vi "Bob.vi"() -> ()   [LabVIEW 2013]
panel:
  in  "Tabs":enum32{"1", "2", "3"}(tab)=enum."2"
  in  "SortearBase":bool
  out "Bases e Estados":string[][](table)=[["", "1", "2", "3", "4", "5", "6", "7", "8", "9", "10", "11", "12", "13", "14", "15", "16", "17", "18", "19", "20"], ["Base", "", "", "", "", "", "", "", "", "", "", "", "", "", "", "", "", "", "", "", ""], ["Estado", "", "", "", "", "", "", "", "", "", "", "", "", "", "", "", "", "", "", "", ""], ["Polarização", "", "", "", "", "", "", "", "", "", "", "", "", "", "", "", "", "", "", "", ""]] caption="Sorteio dos estados para leitura"
  out "Figura":u16(ring)
  in  "MoedaBase":u16(ring)
  in  "Iniciar Calibragem":bool
  in  "Waveform Chart":dbl(graph)
  in  "Coletar medida":bool
  out "Ring":u16(ring) items=["nulo", "nulo", "V", "H", "nulo", "A", "D"]
  in  "ContadorBase":u8=1 min=1
  # "II Semana de Física Experimental"
  # "Criptografia Quântica"
  # "Bob"
  # "Laboratório de Óptica Quântica"
  # "UFRJ"
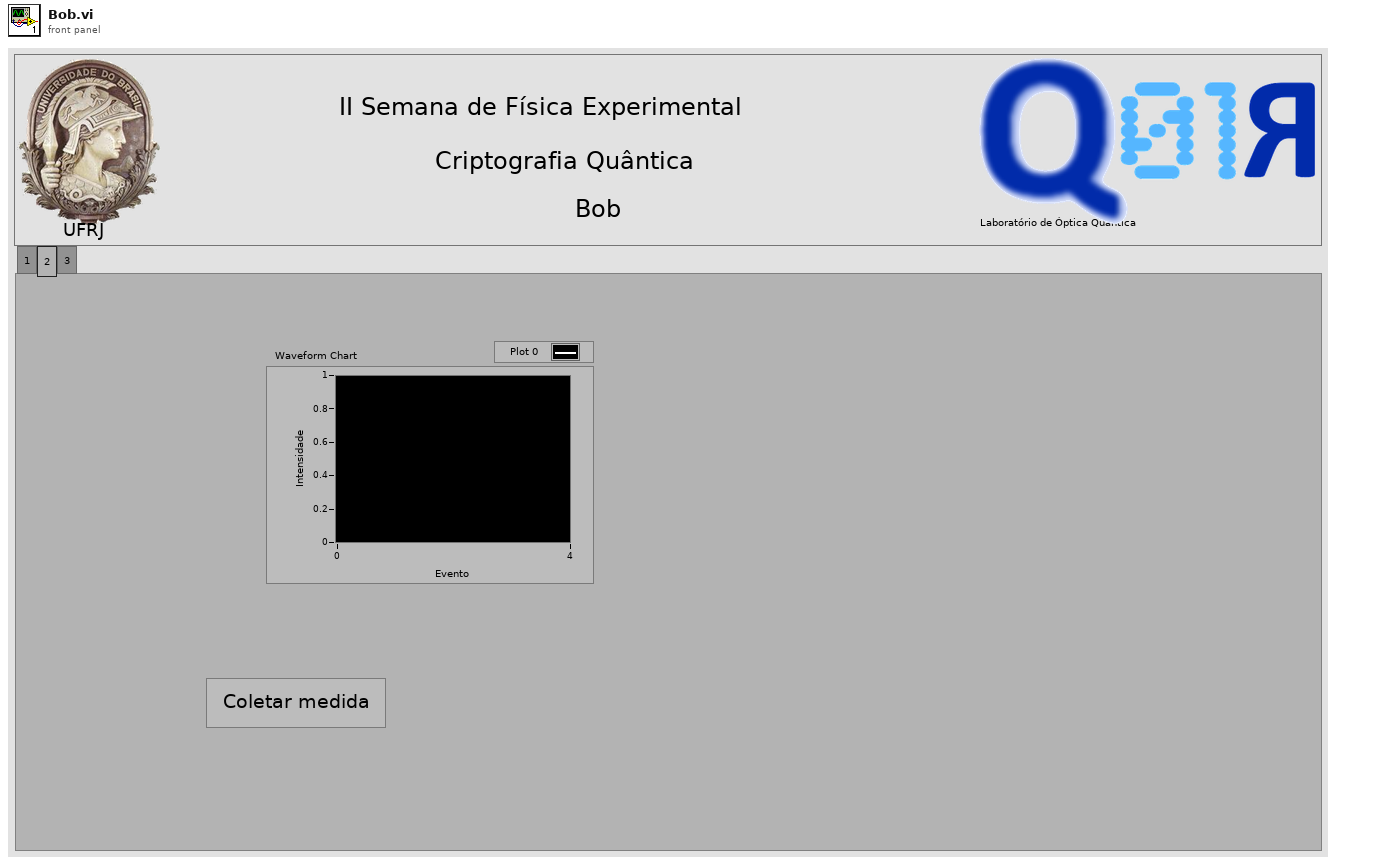
[diagram p1: front panel]
types:
  T1 = enum32{"Page Enabled", "Page Disabled", "Page Disabled & Grayed"}[]
  T2 = enum8{"Enabled", "Disabled", "Disabled and Grayed Out"}
  T3 = enum16{"BCBR", "BC", "BC0", "BC1", "BR", "BR0", "BR1"}
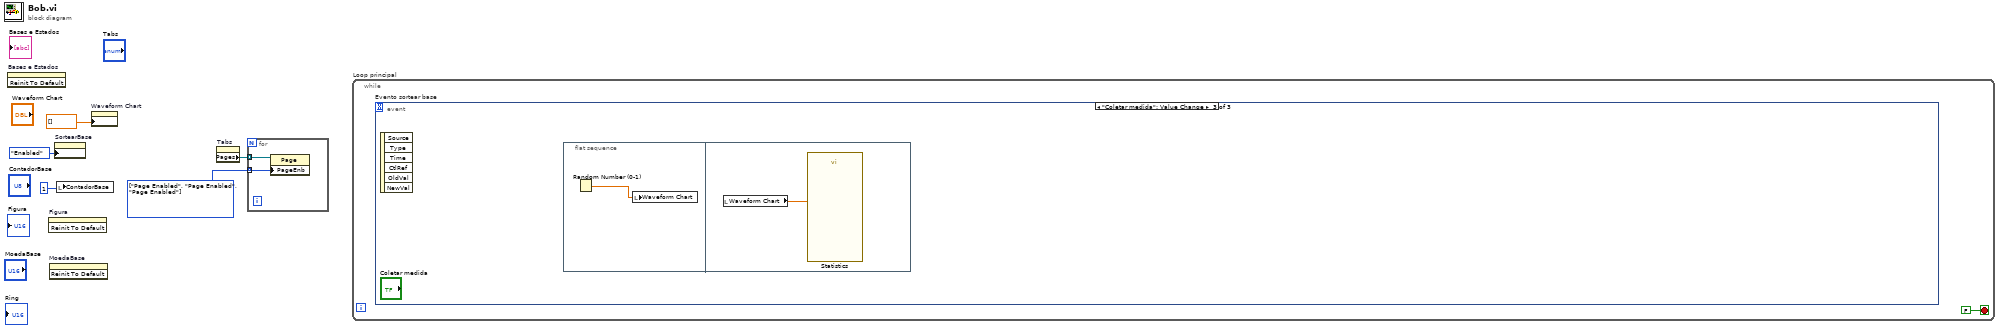
[diagram p0: block diagram]
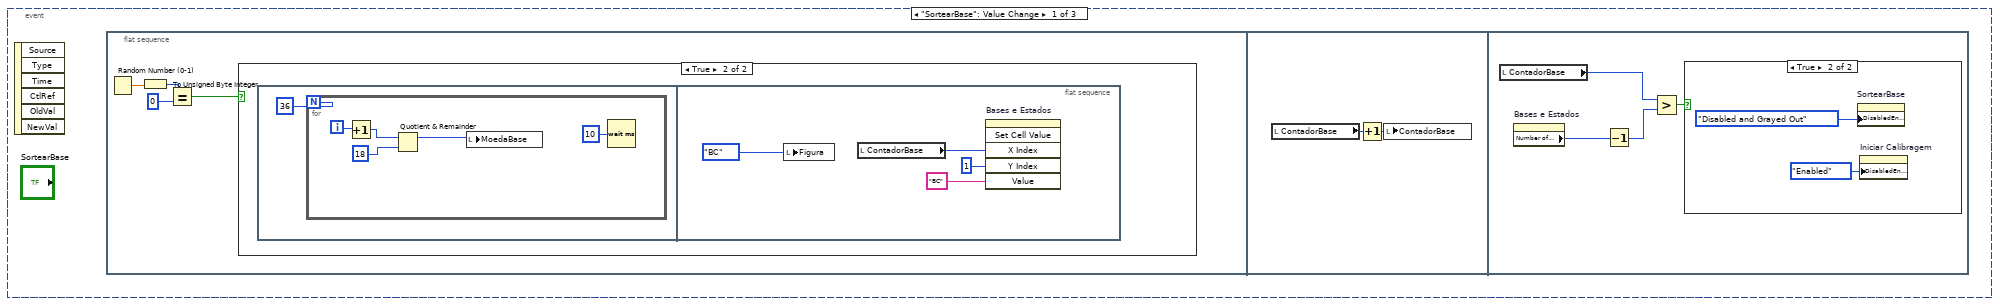
[diagram p2: hidden frame]
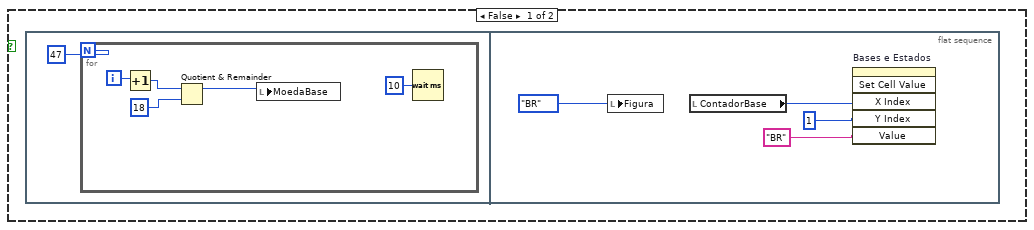
[diagram p3: hidden frame]
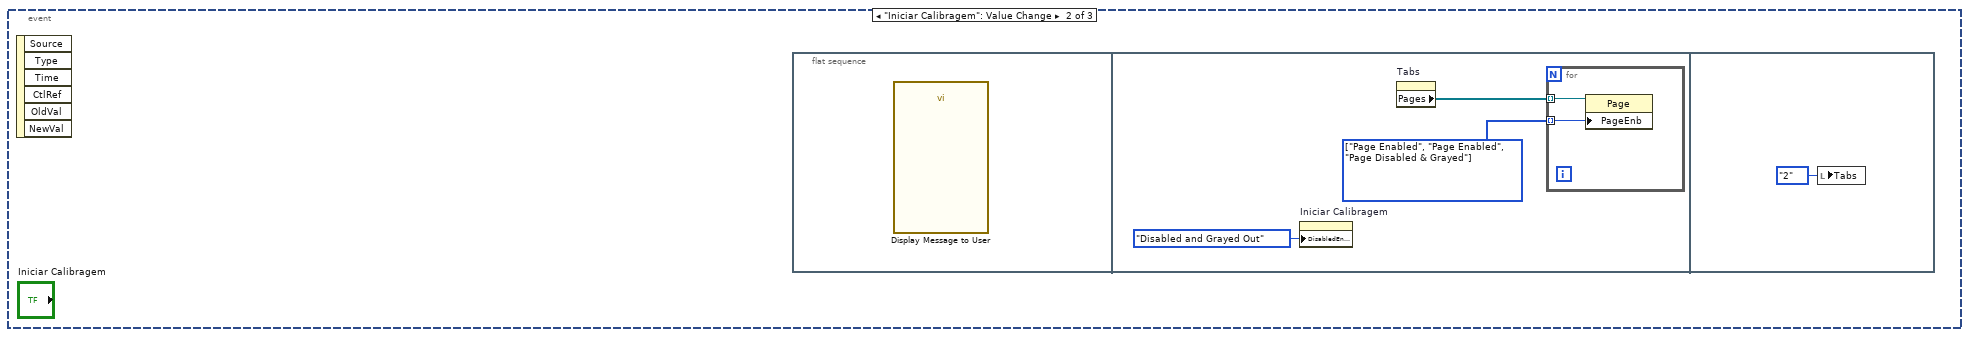
[diagram p5: hidden frame]
diagram:
  w2 = T1 [enum."Page Enabled", enum."Page Enabled", enum."Page Enabled"] items=["Page Enabled", "Page Disabled", "Page Disabled & Grayed"]
  n1 = invoke on="Bases e Estados" class="Tbl (strict)" method="Reinit To Default"() -> ()  [unwired: 3 in, 3 out]
  n2 = invoke on="Figura" class="Ring (strict)" method="Reinit To Default"() -> ()  [unwired: 3 in, 3 out]
  n3 = invoke on="MoedaBase" class="Ring (strict)" method="Reinit To Default"() -> ()  [unwired: 3 in, 3 out]
  n4 = property on="SortearBase" class="Bool"("DisabledEnum"=T2."Enabled" ("Disabled")) -> ()  [unwired: 2 in, 2 out]
  n5 = local write "ContadorBase"(u8 1 ("ContadorBase")) -> ()
  n6 = property on="Waveform Chart" class="WFChart (strict)"("History Data"=dbl[] []) -> ()  [unwired: 2 in, 2 out]
  n7 = property on="Tabs" class="TabCtl (strict)"() -> ("Pages"=w3:refnum<vi>[])  [unwired: 2 in, 2 out]
  n8 = for {
    tunnel: w3 -> [w7] mode=indexing
    tunnel: w2 -> [w6] mode=indexing
    n9 = property class="Page"(reference=w7, "PageEnb"=w6) -> ()  [unwired: 1 in, 2 out]
  }
  n10 = while "Loop principal" {
    stop <- FALSE stop-if-true
    n11 = event "Evento sortear base" shown="[2] \"Coletar medida\": Value Change" {
      selector: _ -> [_ _ _]
      dyn-events: _ -> [_ _ _]
      timeout: _ -> [_ _ _]
      event "SortearBase": Value Change {
        n12 = event-data() -> ()  [unwired: 1 in, 6 out]
        n13 = flat-sequence {
          frame #0 {
            n14 = Random Number (0-1)() -> (number: 0 to 1=w12:dbl)
            n15 = To Unsigned Byte Integer(number=w12) -> (unsigned 8bit integer=w11:u8)
            n16 = Equal?(x=w11, y=u8 0) -> (x = y?=w10:bool)
            n17 = case shown="True" w10 {
              frame False {
                n18 = flat-sequence {
                  frame #0 {
                    n19 = for {
                      N: 47 -> [_]
                      i -> [w14]
                      n20 = Increment(x=w14) -> (x+1=w16:i32)
                      n21 = Quotient & Remainder(x=w16, y=u16 18) -> (x-y*floor(x/y)=w15:i32)  [unwired: 1 out]
                      n22 = local write "MoedaBase"(w15) -> ()
                      n23 = Wait (ms)(milliseconds to wait=u32 10) -> ()  [unwired: 1 out]
                    }
                  }
                  frame #1 {
                    n24 = local write "Figura"(T3."BR") -> ()
                    n25 = local read "ContadorBase"() -> (w21:u8)
                    n26 = invoke on="Bases e Estados" class="Tbl (strict)" method="Set Cell Value"("X Index"=w21, "Y Index"=1, "Value"="BR") -> ()  [unwired: 3 in, 6 out]
                  }
                }
              }
              frame True {
                n27 = flat-sequence {
                  frame #0 {
                    n28 = for {
                      N: 36 -> [_]
                      i -> [w24]
                      n29 = Increment(x=w24) -> (x+1=w26:i32)
                      n30 = Quotient & Remainder(x=w26, y=u16 18) -> (x-y*floor(x/y)=w25:i32)  [unwired: 1 out]
                      n31 = local write "MoedaBase"(w25) -> ()
                      n32 = Wait (ms)(milliseconds to wait=u32 10) -> ()  [unwired: 1 out]
                    }
                  }
                  frame #1 {
                    n33 = local write "Figura"(T3."BC") -> ()
                    n34 = local read "ContadorBase"() -> (w30:u8)
                    n35 = invoke on="Bases e Estados" class="Tbl (strict)" method="Set Cell Value"("X Index"=w30, "Y Index"=1, "Value"="BC" ("String")) -> ()  [unwired: 3 in, 6 out]
                  }
                }
              }
            }
          }
          frame #1 {
            n36 = local read "ContadorBase"() -> (w34:u8)
            n37 = Increment(x=w34) -> (x+1=w33:u8)
            n38 = local write "ContadorBase"(w33) -> ()
          }
          frame #2 {
            n39 = local read "ContadorBase"() -> (w37:u8)
            n40 = property on="Bases e Estados" class="Tbl (strict)"() -> ("Number of Columns"=w38:u32)  [unwired: 2 in, 2 out]
            n41 = Decrement(x=w38) -> (x-1=w36:u32)
            n42 = Greater?(x=w37, y=w36) -> (0:w35:bool)
            n43 = case shown="True" w35 {
              frame False {
              }
              frame True {
                n44 = property on="SortearBase" class="Bool"("DisabledEnum"=T2."Disabled and Grayed Out" ("Disabled")) -> ()  [unwired: 2 in, 2 out]
                n45 = property on="Iniciar Calibragem" class="Bool"("DisabledEnum"=T2."Enabled" ("Disabled")) -> ()  [unwired: 2 in, 2 out]
              }
            }
          }
        }
      }
      event "Iniciar Calibragem": Value Change {
        n46 = event-data() -> ()  [unwired: 1 in, 6 out]
        n47 = flat-sequence {
          frame #0 {
            n48 = call "Display Message to User"() -> ()  [unwired: 10 in, 2 out]
          }
          frame #1 {
            w41 = T1 [enum."Page Enabled", enum."Page Enabled", enum."Page Disabled & Grayed"] items=["Page Enabled", "Page Disabled", "Page Disabled & Grayed"]
            n49 = property on="Iniciar Calibragem" class="Bool"("DisabledEnum"=T2."Disabled and Grayed Out" ("Disabled")) -> ()  [unwired: 2 in, 2 out]
            n50 = property on="Tabs" class="TabCtl (strict)"() -> ("Pages"=w42:refnum<vi>[])  [unwired: 2 in, 2 out]
            n51 = for {
              tunnel: w42 -> [w45] mode=indexing
              tunnel: w41 -> [w44] mode=indexing
              n52 = property class="Page"(reference=w45, "PageEnb"=w44) -> ()  [unwired: 1 in, 2 out]
            }
          }
          frame #2 {
            n53 = local write "Tabs"(enum32{"1", "2", "3"}."2" ("Tabs")) -> ()
          }
        }
      }
      event "Coletar medida": Value Change {
        n54 = event-data() -> ()  [unwired: 1 in, 6 out]
        n55 = flat-sequence {
          frame #0 {
            n56 = Random Number (0-1)() -> (number: 0 to 1=w47:dbl)
            n57 = local write "Waveform Chart"(w47) -> ()
          }
          frame #1 {
            n58 = local read "Waveform Chart"() -> (w48:dbl)
            n59 = call "Statistics"("Signals"=w48) -> ()  [unwired: 21 in, 6 out]
          }
        }
      }
    }
  }
